vi "Pass Object.vi"(0 "LVx.lvlib:LVx.lvclass":refnum<class "LVx.lvclass">, 11 "error in (no error)":errorcluster) -> (15 "error out":errorcluster)   [LabVIEW 2011, in "LVx.lvlib" / "LVx.lvclass"]
uses:
  LVx.lvclass
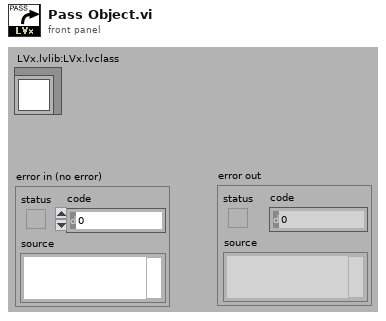
[diagram p1: front panel]
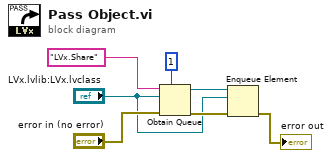
[diagram p0: block diagram]
diagram:
  n1 = Obtain Queue(max queue size (-1, unlimited)=1, name (unnamed)="LVx.Share", element data type="LVx.lvlib:LVx.lvclass", error in (no error)="error in (no error)") -> (queue out=w3:refnum<queue>, error out=w4:errorcluster)  [unwired: 1 in, 1 out]
  n2 = Enqueue Element(queue=w3, element="LVx.lvlib:LVx.lvclass", error in (no error)=w4) -> (error out=→"error out":errorcluster)  [unwired: 3 out]
